vi "dfd_Maxflat Domain Conversion.vi"(4 "N":i32=2, 6 "M":i32=1, 7 "symmetric FIR ? (T)":bool, 8 "error in (no error)":errorcluster, 9 "c":dbl, 10 "denominator":dbl[](array[numeric]), 11 "numerator":dbl[](array[numeric]) format="%_10g") -> (0 "error out":errorcluster, 2 "poles":cdb[](array[numeric]), 3 "zeros":cdb[](array[numeric]) format="%#_6e")   [LabVIEW 2017, in "NI_DigFilter_Design.lvlib"]
doc: "Converts the <B>numerator</B> and <B>denominator</B> of the polynomial to z domain."
uses:
  <vilib>/addons/Digital Filter Design/NI_DigFilter_Design.lvlib
  <vilib>/addons/Digital Filter Design/_Misc.llb/dfd_Error Cluster From Error Code (Scalar).vi
  <vilib>/addons/Digital Filter Design/_Misc.llb/dfd_Error Handlers (Single).vi
  <vilib>/addons/Digital Filter Design/NI_DigFilterLicensed.lvlib
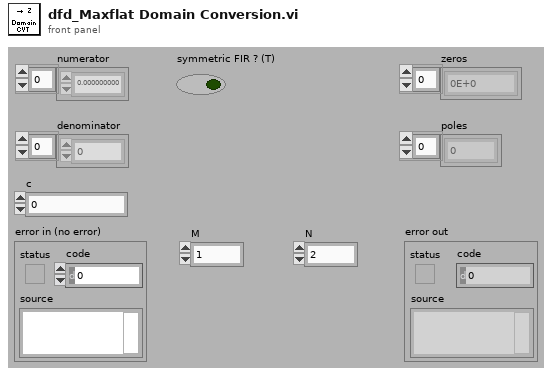
[diagram p1: front panel]
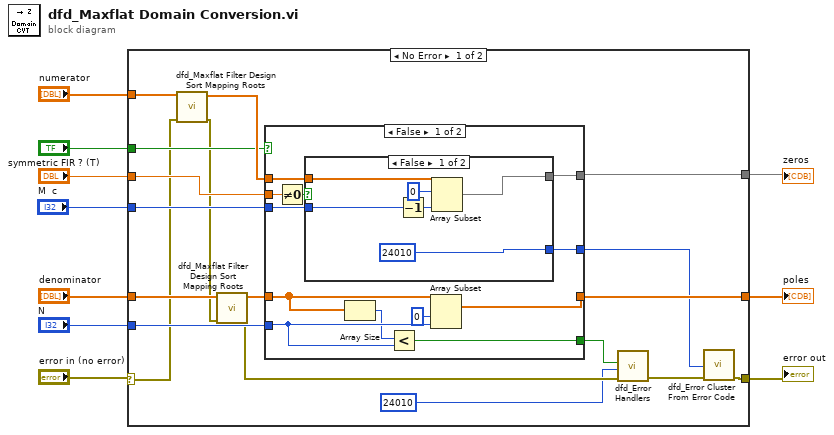
[diagram p0: block diagram]
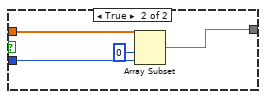
[diagram p2: hidden frame]
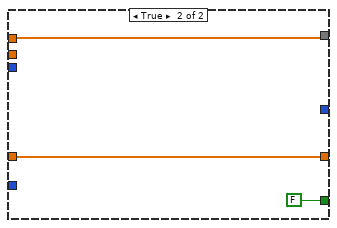
[diagram p3: hidden frame]
diagram:
  n1 = case shown="No Error" "error in (no error)" {
    selector: "error in (no error)" -> [w19 w54]
    tunnel: "N" -> [w28 _]
    tunnel: "denominator" -> [w26 _]
    tunnel: "numerator" -> [w24 _]
    tunnel: "M" -> [w23 _]
    tunnel: "c" -> [w22 _]
    tunnel: "symmetric FIR ? (T)" -> [w21 _]
    tunnel: [w17 _] -> w4
    tunnel: [w18 _] -> w3
    tunnel: [w15 w54] -> w2
    frame No Error {
      n2 = call <vilib>:"dfd_Maxflat Filter Design Sort Mapping Roots.vi"("error in (no error)"=w19, "polynomial"=w24) -> ("error out"=w20:errorcluster, "roots"=w25:cdb[])  [unwired: 8 out]
      n3 = call <vilib>:"dfd_Maxflat Filter Design Sort Mapping Roots.vi"("error in (no error)"=w20, "polynomial"=w26) -> ("error out"=w16:errorcluster, "roots"=w27:cdb[])  [unwired: 8 out]
      n4 = case shown="False" w21 {
        tunnel: w22 -> [w40 _]
        tunnel: w23 -> [w38 _]
        tunnel: w25 -> [w37 w53]
        tunnel: w27 -> [w31 w52]
        tunnel: w28 -> [w32 _]
        tunnel: [w35 w53] -> w17
        tunnel: [w34 w52] -> w18
        tunnel: [w33 _] -> w14
        tunnel: [w29 FALSE] -> w12
        frame False {
          n5 = Not Equal To 0?(x=w40) -> (x != 0?=w39:bool)
          n6 = case shown="False" w39 {
            tunnel: w37 -> [w45 w48]
            tunnel: w38 -> [w44 w49]
            tunnel: [w42 w47] -> w35
            tunnel: [24010 ("WRN_ORDER_BE_LOWER") _] -> w33
            frame False {
              n7 = Decrement(x=w44) -> (x-1=w43:i32)
              n8 = Array Subset(array=w45, index=0, length=w43) -> (w42:cdb[])
            }
            frame True {
              n9 = Array Subset(array=w48, index=0, length=w49) -> (w47:cdb[])
            }
          }
          n10 = Array Size(array=w31) -> (size(s)=w30:i32)
          n11 = Less?(x=w30, y=w32) -> (x < y?=w29:bool)
          n12 = Array Subset(array=w31, index=0, length=w32) -> (w34:cdb[])
        }
        frame True {
        }
      }
      n13 = call-poly <vilib>:"dfd_Error Handlers.vi"("error in (no error)"=w16, "error code"=24010 ("WRN_ORDER_BE_LOWER"), "condition failed?"=w12) -> ("error out"=w13:errorcluster)  [unwired: 8 out]
      n14 = call-poly <vilib>:"dfd_Error Cluster From Error Code.vi"("error in (no error)"=w13, "error code (0)"=w14) -> ("error out"=w15:errorcluster)  [unwired: 9 out]
    }
    frame Error {
    }
  }
  "poles" <- w3
  "zeros" <- w4
  "error out" <- w2
